vi "Load .Obj File.vi"(5 "Load Material Textures (Default: True)":bool=TRUE, 6 "Material Search Folder (Default: Empty - Use Model Path Folder)":path, 7 "Force Regenerate Normals (Defaut: False)":bool, 8 "error in (no error)":errorcluster, 11 "Object Model Path":path) -> (0 "error out":errorcluster, 3 "Objects":refnum<vi>[](array[refnum]), 4 "Bounding Box":T1)   [LabVIEW 2020, in "g_ar_toolkit.ar.lvlib"]
uses:
  g_ar_toolkit.ar.lvlib
  Model Bounding Box.ctl
  g_ar_toolkit.common/Object Point (Float).ctl
  Vertex Descriptor.ctl
  <vilib>/Utility/miscctls.llb/LV3DPointTypeDef.ctl
  <vilib>/picture/3D Picture Control/Geometries/Create Mesh.vi
  <vilib>/picture/3D Picture Control/Object/Create Object.vi
  <vilib>/picture/3D Picture Control/Object/Create Object (drawable).vi
  <vilib>/picture/3D Picture Control/Object/Set Material.vi
  <vilib>/Utility/libraryn.llb/Get File Extension.vi
  <vilib>/picture/jpeg.llb/Read JPEG File.vi
  <vilib>/picture/3D Picture Control/Helpers/Apply Texture.vi
  <vilib>/picture/3D Picture Control/Helpers/Apply Texture (no reference).vi
  <vilib>/picture/png.llb/Read PNG File.vi
  <vilib>/picture/bmp.llb/Read BMP File.vi
  bin/g_ar_toolkit.1.32.dll
  g_ar_toolkit.common/g_ar_toolkit.common.lvlib
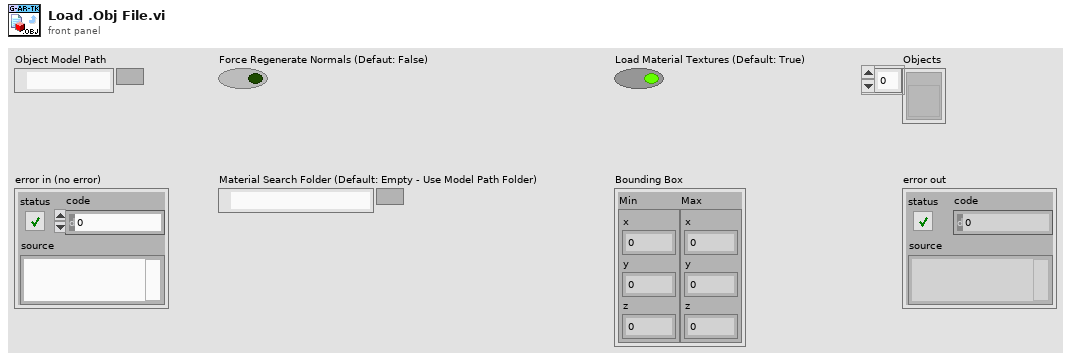
[diagram p1: front panel]
types:
  T1 = typedef "g_ar_toolkit.ar.lvlib/Model Bounding Box.ctl" = cluster{"Min":T2, "Max":T2}
  T2 = typedef "g_ar_toolkit.common.lvlib/Object Point (Float).ctl" = cluster{"x":dbl, "y":dbl, "z":dbl}
  T3 = typedef "g_ar_toolkit.ar.lvlib/Vertex Descriptor.ctl" = cluster{"Vertex":T4, "Normal":T4, "Colour":cluster{"R":sgl, "G":sgl, "B":sgl}, "Texture Coord":cluster{"S":sgl, "T":sgl}}
  T4 = typedef "LV3DPointTypeDef.ctl" = cluster{"X":sgl, "Y":sgl, "Z":sgl}
  T5 = cluster{"Name":string, "Shininess":sgl, "Ambient":cluster{"Red":sgl, "Green":sgl, "Blue":sgl}, "Specular":cluster{"Red":sgl, "Green":sgl, "Blue":sgl}, "Emission":cluster{"Red":sgl, "Green":sgl, "Blue":sgl}, "Diffuse":cluster{"Red":sgl, "Green":sgl, "Blue":sgl}, "texture-name":string}[]
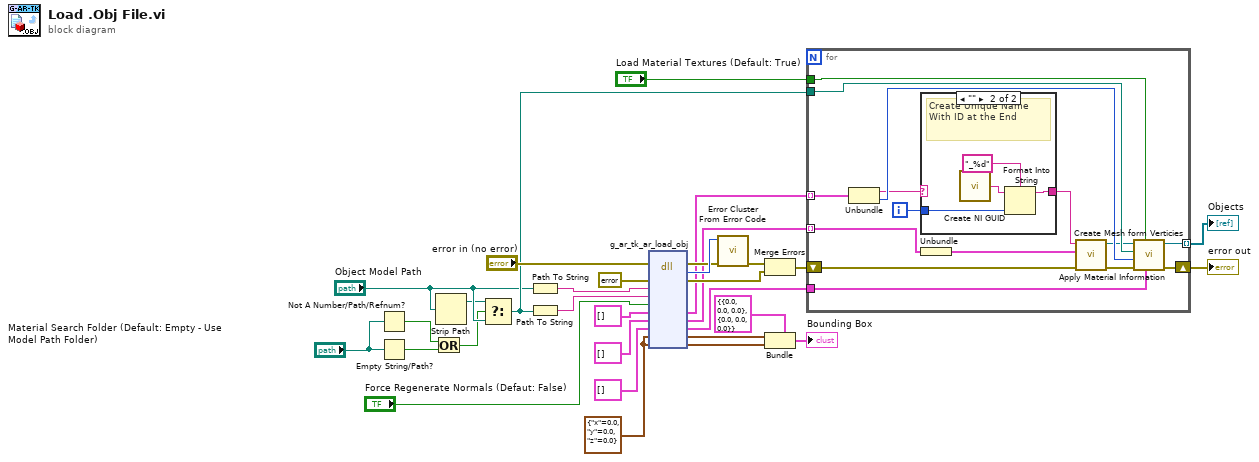
[diagram p0: block diagram]
diagram:
  w22 = T2 {"x"=0.0, "y"=0.0, "z"=0.0} ("Object Point")
  n1 = Not A Number/Path/Refnum?(number/path/refnum="Material Search Folder (Default: Empty - Use Model Path Folder)") -> (NaN/Path/Refnum?=w7:bool)
  n2 = Empty String/Path?(string/path="Material Search Folder (Default: Empty - Use Model Path Folder)") -> (empty?=w1:bool)
  n3 = Or(x=w7, y=w1) -> (x .or. y?=w2:bool)
  n4 = Strip Path(path="Object Model Path") -> (stripped path=w4:path)  [unwired: 1 out]
  n5 = Select(t=w4, s=w2, f="Object Model Path") -> (s? t:f=w6:path)
  n6 = Path To String(path="Object Model Path") -> (string=w21:string)
  n7 = Path To String(path=w6) -> (string=w20:string)
  n8 = dll-call lib="C:/serenial/libraries/g-augmented-reality-toolkit/LabVIEW/bin/g_ar_toolkit.1.*.*" fn="g_ar_tk_ar_load_obj" ("g_ar_toolkit.*.*:g_ar_tk_image_copy")(error in="error in (no error)", "error_cluster"=errorcluster {"status"=FALSE, "code"=0, "source"=""} ("error constant"), "object_path"=w21, "material_path"=w20, "regen_normals"="Force Regenerate Normals (Defaut: False)", "object_array"=cluster{"name":string, "material_id":i32}[] [], "point_arrays"=cluster{"Verticies":T3[]}[] [], "material_array"=T5 [] ("Materials"), "bbox_min"=w22, "bbox_max"=w22) -> (error out=w26:errorcluster, "MgErr"=w27:i32, "error_cluster"=w30:errorcluster, "object_array"=w18:cluster{"name":string, "material_id":i32}[], "point_arrays"=w14:cluster{"Verticies":T3[]}[], "material_array"=w13:T5, "bbox_min"=w11:T2, "bbox_max"=w10:T2)  [unwired: 5 in, 1 out]
  n9 = call <vilib>:"Error Cluster From Error Code.vi"("error in (no error)"=w26, "error code (0)"=w27) -> ("error out"=w28:errorcluster)  [unwired: 7 in]
  n10 = Merge Errors(w28, w30) -> (w19:errorcluster)
  n11 = Bundle(cluster=T1 {"Min"={"x"=0.0, "y"=0.0, "z"=0.0}, "Max"={"x"=0.0, "y"=0.0, "z"=0.0}} ("Bounding Box"), "Min"=w11, "Max"=w10) -> (→"Bounding Box":T1)
  n12 = for {
    tunnel: w18 -> [w46] mode=indexing
    tunnel: [w45] -> w17 mode=indexing
    tunnel: w13 -> [w43]
    shift-right: [w44] -> w16
    shift-left: w19 -> [w42]
    tunnel: w6 -> [w40]
    tunnel: w14 -> [w36] mode=indexing
    tunnel: "Load Material Textures (Default: True)" -> [w32]
    i -> [w38]
    n13 = Unbundle(w46) -> ("name"=w39:string, "material_id"=w41:i32)
    n14 = case shown="\"\"" w39 {
      selector: w39 -> [w47 _]
      tunnel: w38 -> [_ w51]
      tunnel: [w47 w48] -> w37
      frame Default {
      }
      frame "" {
        # "Create Unique Name With ID at the End"
        n15 = call <vilib>:"Create NI GUID.vi"() -> ("NI GUID"=w50:string)
        n16 = Format Into String(format string="_%d", initial string=w50, w51) -> (resulting string=w48:string)  [unwired: 1 in, 1 out]
      }
    }
    n17 = Unbundle(w36) -> ("Verticies"=w35:T3[])
    n18 = call "Create Mesh form Verticies.vi"("error in (no error)"=w42, "Verticies"=w35, "Object Name"=w37) -> ("error out"=w33:errorcluster, "SceneObject out"=w34:refnum<vi>)  [unwired: 7 in]
    n19 = call "Apply Material Information.vi"("Materials"=w43, "Load Material Textures"=w32, "error in (no error)"=w33, "material_id"=w41, "Material Path"=w40, "SceneObject in"=w34) -> ("error out"=w44:errorcluster, "SceneObject out"=w45:refnum<vi>)  [unwired: 4 in]
  }
  "Objects" <- w17
  "error out" <- w16
